vi "Drive Distance.vi"(10 "Desired Right Inches":dbl, 11 "Desired Left Inches":dbl) -> ()   [LabVIEW 2014]
uses:
  <vilib>/Rock Robotics/WPI/Solenoid/WPI_SolenoidValue.ctl
  <vilib>/Rock Robotics/WPI/Solenoid/WPI_SolenoidSetEnum.vi
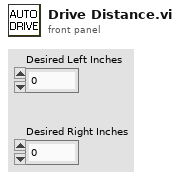
[diagram p1: front panel]
types:
  T1 = typedef "WPI_EncoderDevRef.ctl" = cluster{"DevStatus":errorcluster, "EncoderIndex":T2, "CounterIndex":T3, "DistancePerCount":dbl, "Decoding Type":T4}
  T2 = typedef "FPGA_EncoderIdx.ctl" = enum8{"Enc 0", "Enc 1", "Enc 2", "Enc 3", "Enc 4", "Enc 5", "Enc 6", "Enc 7", "Invalid"}
  T3 = typedef "FPGA_CounterCtrSystemIndex.ctl" = enum8{"Ctr 0", "Ctr 1", "Ctr 2", "Ctr 3", "Ctr 4", "Ctr 5", "Ctr 6", "Ctr 7", "Invalid"}
  T4 = typedef "WPI_EncoderType.ctl" = enum16{"1x", "2x", "4x"}
  T5 = typedef "WPI_SolenoidValue.ctl" = enum16{"Off", "On", "Forward", "Reverse"}
  T6 = typedef "WPI_GyroDevRef.ctl" = cluster{"DevStatus":errorcluster, "Analog Module":T7, "Analog Channel":T8, "Offset":dbl, "Gain (VoltsPerDegree/Second)":dbl}
  T7 = typedef "FPGA_TypedefAnalogModule.ctl" = enum16{"Controller 1"}
  T8 = typedef "FPGA_AIChannel.ctl" = enum8{"AI 0", "AI 1", "AI 2", "AI 3", "AI MXP 0", "AI MXP 1", "AI MXP 2", "AI MXP 3", "Invalid"}
  T9 = typedef "WPI_SolenoidDevRef.ctl" = cluster{"DevStatus":errorcluster, "Pneumatics Control Module":u8, "Forward Solenoid Channel":T10, "Reverse Solenoid Channel":T10}
  T10 = typedef "WPI_SolenoidChannel.ctl" = enum8{"Solenoid 0", "Solenoid 1", "Solenoid 2", "Solenoid 3", "Solenoid 4", "Solenoid 5", "Solenoid 6", "Solenoid 7", "Invalid"}
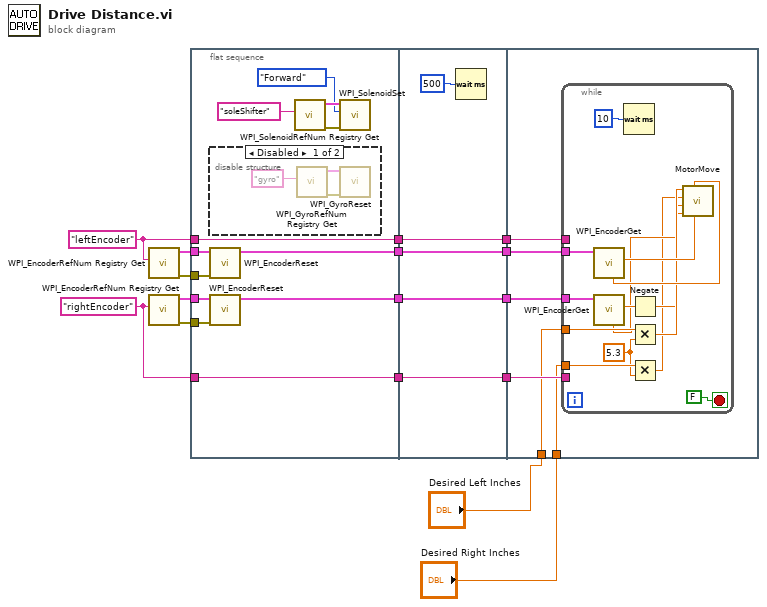
[diagram p0: block diagram]
diagram:
  w11 = "rightEncoder" ("refnum name")
  w12 = "leftEncoder" ("refnum name")
  n1 = call <vilib>:"WPI_EncoderRefNum Registry Get.vi"("refnum name"=w12) -> ("error out"=w15:errorcluster, "EncoderDevRef"=w16:T1)  [unwired: 9 in]
  n2 = call <vilib>:"WPI_EncoderRefNum Registry Get.vi"("refnum name"=w11) -> ("error out"=w13:errorcluster, "EncoderDevRef"=w14:T1)  [unwired: 9 in]
  n3 = flat-sequence {
    tunnel: w16 -> [w28]
    tunnel: w15 -> [w27]
    tunnel: w14 -> [w26]
    tunnel: w13 -> [w25]
    tunnel: w12 -> [w24]
    tunnel: [w24] -> w10
    tunnel: w11 -> [w21]
    tunnel: [w21] -> w8
    tunnel: [w23] -> w6
    tunnel: [w22] -> w4
    tunnel: w10 -> [w36]
    tunnel: [w36] -> w9
    tunnel: w8 -> [w35]
    tunnel: [w35] -> w7
    tunnel: w6 -> [w34]
    tunnel: [w34] -> w5
    tunnel: w4 -> [w33]
    tunnel: [w33] -> w3
    tunnel: w9 -> [w42]
    tunnel: w7 -> [w41]
    tunnel: "Desired Left Inches" -> [w40]
    tunnel: "Desired Right Inches" -> [w39]
    tunnel: w5 -> [w38]
    tunnel: w3 -> [w37]
    frame #0 {
      n4 = disable-structure shown="Disabled" {
        frame Disabled {
          n5 = call <vilib>:"WPI_GyroRefNum Registry Get.vi"("refnum name"="gyro") -> ("error out"=w30:errorcluster, "GyroDevRef"=w31:T6)  [unwired: 9 in]
          n6 = call <vilib>:"WPI_GyroReset.vi"("error in (no error)"=w30, "GyroDevRef"=w31) -> ()  [unwired: 8 in, 2 out]
        }
        frame Enabled {
        }
      }
      n7 = call <vilib>:"WPI_EncoderReset.vi"("error in (no error)"=w27, "EncoderDevRef"=w28) -> ("EncoderDevRef"=w23:T1)  [unwired: 8 in, 1 out]
      n8 = call <vilib>:"WPI_EncoderReset.vi"("error in (no error)"=w25, "EncoderDevRef"=w26) -> ("EncoderDevRef"=w22:T1)  [unwired: 8 in, 1 out]
      n9 = call <vilib>:"WPI_SolenoidRefNum Registry Get.vi"("refnum name"="soleShifter") -> ("error out"=w19:errorcluster, "SolenoidDevRef"=w20:T9)  [unwired: 9 in]
      n10 = call-poly <vilib>:"WPI_SolenoidSet.vi"("error in (no error)"=w19, "Value"=WPI_SolenoidValue."Forward", "SolenoidDevRef"=w20) -> ()  [unwired: 7 in, 2 out]
    }
    frame #1 {
      n11 = Wait (ms)(milliseconds to wait=u32 500) -> ()  [unwired: 1 out]
    }
    frame #2 {
      n12 = while {
        tunnel: w42 -> [_]
        tunnel: w41 -> [_]
        tunnel: w40 -> [w56]
        tunnel: w39 -> [w55]
        tunnel: w38 -> [w51]
        tunnel: w37 -> [w50]
        stop <- FALSE stop-if-true
        w54 = 5.3 ("y")
        n13 = call <vilib>:"WPI_EncoderGet.vi"("EncoderDevRef"=w51) -> ("Distance"=w48:dbl, "Rate"=w47:dbl)  [unwired: 5 in, 4 out]
        n14 = call <vilib>:"WPI_EncoderGet.vi"("EncoderDevRef"=w50) -> ("Distance"=w49:dbl, "Rate"=w44:dbl)  [unwired: 5 in, 4 out]
        n15 = Wait (ms)(milliseconds to wait=u32 10) -> ()  [unwired: 1 out]
        n16 = Negate(x=w49) -> (-x=w45:dbl)
        n17 = Multiply(x=w56, y=w54) -> (x*y=w46:dbl)
        n18 = Multiply(x=w55, y=w54) -> (x*y=w43:dbl)
        n19 = call "MotorMove.vi"("Left Encoder Distance"=w48, "Left Rate"=w47, "Right Rate"=w44, "Right Encoder Distance"=w45, "Right Desired"=w43, "Left Desired"=w46) -> ()  [unwired: 6 in]
      }
    }
  }
